vi "update_faux_worm_positions.vi"(3 "Update Time (ms)":sgl, 5 "Worms to Draw":T1[](array[typedef])) -> (2 "Worms to Draw Updated":T1[](array[typedef]))   [LabVIEW 2019]
uses:
  FauxWorm.ctl
  ParametersGlobal.vi
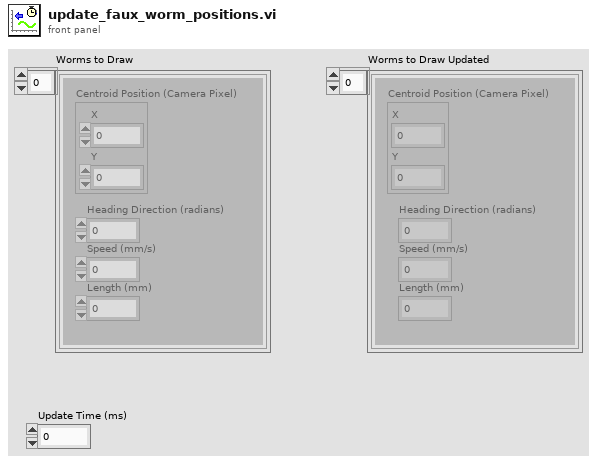
[diagram p1: front panel]
types:
  T1 = typedef "FauxWorm.ctl" = cluster{"Centroid Position (Camera Pixel)":cluster{"X":sgl, "Y":sgl}, "Heading Direction (radians)":dbl, "Speed (mm/s)":sgl, "Length (mm)":sgl}
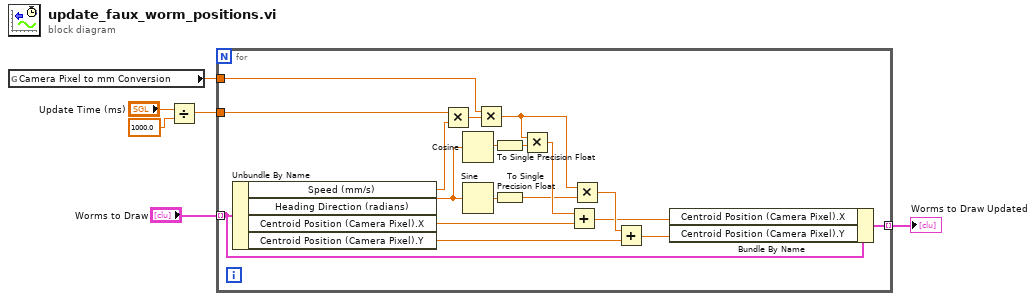
[diagram p0: block diagram]
diagram:
  n1 = global read "ParametersGlobal.vi" "Camera Pixel to mm Conversion"() -> (w4:sgl)
  n2 = Divide(x="Update Time (ms)", y=sgl 1000.0) -> (x/y=w2:sgl)
  n3 = for {
    tunnel: "Worms to Draw" -> [w16] mode=indexing
    tunnel: [w13] -> w5 mode=indexing
    tunnel: w4 -> [w12]
    tunnel: w2 -> [w7]
    n4 = Unbundle By Name(w16) -> ("Speed (mm/s)"=w24:sgl, "Heading Direction (radians)"=w22:dbl, "Centroid Position (Camera Pixel).X"=w21:sgl, "Centroid Position (Camera Pixel).Y"=w18:sgl)
    n5 = Multiply(x=w7, y=w24) -> (x*y=w23:sgl)
    n6 = Cosine(x=w22) -> (cos(x)=w11:dbl)
    n7 = Sine(x=w22) -> (sin(x)=w9:dbl)
    n8 = Multiply(x=w12, y=w23) -> (x*y=w20:sgl)
    n9 = To Single Precision Float(number=w11) -> (single precision float=w10:sgl)
    n10 = To Single Precision Float(number=w9) -> (single precision float=w8:sgl)
    n11 = Multiply(x=w20, y=w10) -> (x*y=w19:sgl)
    n12 = Add(x=w19, y=w21) -> (x+y=w14:sgl)
    n13 = Multiply(x=w20, y=w8) -> (x*y=w17:sgl)
    n14 = Add(x=w17, y=w18) -> (x+y=w15:sgl)
    n15 = Bundle By Name(cluster=w16, "Centroid Position (Camera Pixel).X"=w14, "Centroid Position (Camera Pixel).Y"=w15) -> (w13:T1)
  }
  "Worms to Draw Updated" <- w5
